vi "Set Rate (RPM).vi"(8 "error in (no error)":errorcluster, 10 "Rate (RPM)":dbl, 11 "Comp Motors with Encoders in":refnum<class "Comp Motors with Encoders.lvclass">) -> (0 "error out":errorcluster, 3 "Comp Motors with Encoders out":refnum<class "Comp Motors with Encoders.lvclass">)   [LabVIEW 2014, in "Comp Motors with Encoders.lvlib" / "Comp Motors with Encoders.lvclass"]
uses:
  Comp Motors with Encoders.lvclass
  Comp Motors with Encoders.lvclass/Comp Motors with Encoders.ctl
  Robot/Motor with Encoders/Motors with Encoders Class/Motors with Encoders.lvclass
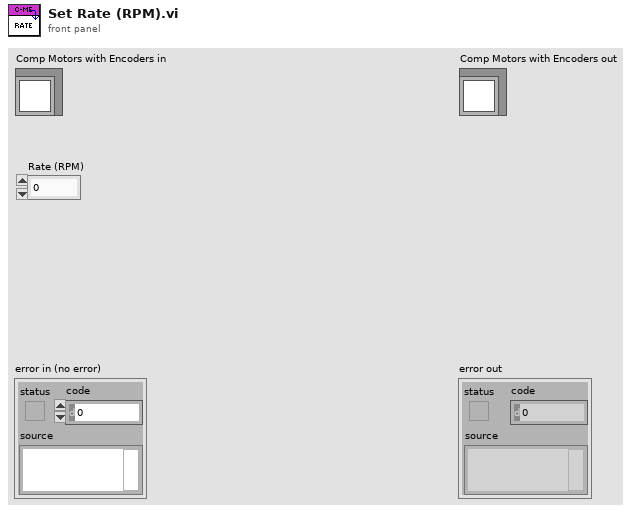
[diagram p1: front panel]
types:
  T1 = enum16{"Critical", "Error", "Warning", "Informational", "Debug"}
  T2 = typedef "WPI_MotorControlDeviceRef.ctl" = cluster{"DeviceStatus":errorcluster, "Type":T3, "PWM":cluster{"Controller":T4, "PWM Channel":T5, "DeadBand":T6}, "CAN":cluster{"Device Number":u8, "Control Mode":T7, "Semaphore":T8, "Max Vout":dbl, "TalonSRX Control Mode":T9}, "Invert":bool, "TransformRef":T10, "InvTransformRef":T10}
  T3 = typedef "WPI_MotorControlType.ctl" = enum16{"PWM", "CAN", "CANTalonSRX"}
  T4 = typedef "FPGA_TypedefDigitalModule.ctl" = enum16{"Controller 1"}
  T5 = typedef "FPGA_DIOPWMChannel.ctl" = enum8{"PWM 0", "PWM 1", "PWM 2", "PWM 3", "PWM 4", "PWM 5", "PWM 6", "PWM 7", "PWM 8", "PWM 9", "PWM MXP 0", "PWM MXP 1", "PWM MXP 2", "PWM MXP 3", "PWM MXP 4", "PWM MXP 5", "PWM MXP 6", "PWM MXP 7", "PWM MXP 8", "PWM MXP 9", "Invalid"}
  T6 = typedef "WPI_PWMDeadband.ctl" = cluster{"Name":string, "maxPositivePwm":i32, "minPositivePwm":i32, "centerPwm":i32, "maxNegativePwm":i32, "minNegativePwm":i32, "angularRange":u16}
  T7 = typedef "WPI_CANJaguar_ControlMode.ctl" = enum8{"Percent VBus", "Current", "Speed", "Position", "Voltage"}
  T8 = typedef "Semaphore RefNum" = refnum<k1>
  T9 = typedef "WPI_CANTalonSRX_APIControlMode.ctl" = enum8{"Percent VBus", "Speed", "Position", "Slave", "Unchanged / Invalid"}
  T10 = typedef "WPI_PWMTransform_ConPane.ctl" = refnum<vi>
  T11 = typedef "Motors with Encoders.lvlib/Motors with Encoders.lvclass/Motors with Encoders State.ctl" = cluster{"Forward Switch":bool, "Reverse Switch":bool, "Measured RPM":dbl, "Distance (in)":dbl, "Setpoint RPM":dbl, "Encoder Count":i64, "Home Count":i64, "Config":T12}
  T12 = typedef "Motors with Encoders.lvlib/Motors with Encoders.lvclass/Motors with Encoders Config.ctl" = cluster{"Counts  Per Revolution":u32, "Invert Encoder Direction":bool, "Diameter of Revolution":dbl, "Max RPM":dbl, "Encoder Control":bool}
  T13 = typedef "WPI_CANTalonSRX_GlobalStatus.ctl" = cluster{"Applied Throttle":dbl, "Module Enabled":bool, "CAN Error":errorcluster, "Closed Loop Error":dbl, "Forward Limit Switch Closed":bool, "Reverse Limit Switch Closed":bool, "Sensor Position":dbl, "Sensor Velocity":dbl, "Current":dbl, "Sticky Fault - Over Temp":bool, "Sticky Fault - Under Voltage":bool, "Sticky Fault - Forward Limit":bool, "Sticky Fault - Reverse Limit":bool, "Sticky Fault - Forward Soft Limit":bool, "Sticky Fault - Reverse Soft Limit":bool, "Brake is Enabled":bool, "Encoder Position":dbl, "Encoder Velocity":dbl, "Encoder Index Count":dbl, "Encoder A Pin State":bool, "Encoder B Pin State":bool, "Encoder Index Pin State":bool, "Analog In":dbl, "Analog In Velocity":dbl, "Temperature (C)":dbl, "Battery Voltage":dbl}
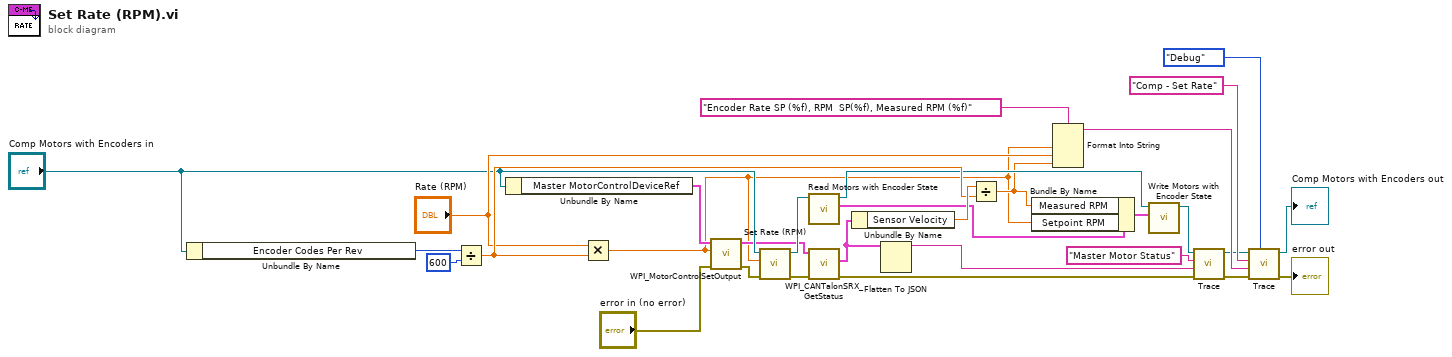
[diagram p0: block diagram]
diagram:
  n1 = Unbundle By Name("Comp Motors with Encoders in") -> ("Encoder Codes Per Rev"=w17:u16)
  n2 = Divide(x=w17, y=u16 600) -> (x/y=w13:dbl)
  n3 = Unbundle By Name("Comp Motors with Encoders in") -> ("Master MotorControlDeviceRef"=w30:T2)
  n4 = Multiply(x="Rate (RPM)", y=w13) -> (x*y=w1:dbl)
  n5 = call <vilib>:"WPI_MotorControlSetOutput.vi"("error in (no error)"="error in (no error)", "Output"=w1, "MotorControlDevRef"=w30) -> ("error out"=w2:errorcluster, "MotorControlDevRef"=w3:T2)  [unwired: 6 in, 1 out]
  n6 = call-parent "Set Rate (RPM).vi"("error in (no error)"=w2, "Rate (RPM)"=w1, "Motors with Encoders in"="Comp Motors with Encoders in") -> ("error out"=w23:errorcluster, "Motors with Encoders out"=w12:refnum<class "Comp Motors with Encoders.lvclass">)  [unwired: 7 in]
  n7 = call-dynamic "Read Motors with Encoder State.vi"("Motors with Encoders in"=w12) -> ("Motors with Encoder State"=w9:T11, "Motors with Encoders out"=w11:refnum<class "Comp Motors with Encoders.lvclass">)  [unwired: 8 in, 1 out]
  n8 = call <vilib>:"WPI_CANTalonSRX_GetStatus.vi"("error in (no error)"=w23, "CAN Talon SRX Ref"=w3) -> ("error out"=w22:errorcluster, "Talon SRX Status"=w15:T13)  [unwired: 7 in, 1 out]
  n9 = Unbundle By Name(w15) -> ("Sensor Velocity"=w14:dbl)
  n10 = Flatten To JSON(anything=w15) -> (JSON string=w19:string)  [unwired: 2 in, 1 out]
  n11 = Divide(x=w14, y=w13) -> (x/y=w7:dbl)
  n12 = Bundle By Name(cluster=w9, "Measured RPM"=w7, "Setpoint RPM"=w1) -> (w8:T11)
  n13 = Format Into String(format string="Encoder Rate SP (%f), RPM  SP(%f), Measured RPM (%f)", w1, "Rate (RPM)", w7) -> (resulting string=w24:string)  [unwired: 2 in, 1 out]
  n14 = call-dynamic "Write Motors with Encoder State.vi"("Motors with Encoder State"=w8, "Motors with Encoders in"=w11) -> ("Motors with Encoders out"=w10:refnum<class "Comp Motors with Encoders.lvclass">)  [unwired: 8 in, 1 out]
  n15 = call-dynamic "Trace.vi"("error in (no error)"=w22, "System Message"=w19, "System Action"="Master Motor Status", "System Actor in"=w10) -> ("error out"=w21:errorcluster, "System Actor out"=w20:refnum<class "Comp Motors with Encoders.lvclass">)  [unwired: 6 in]
  n16 = call-dynamic "Trace.vi"("Trace Level"=T1."Debug", "error in (no error)"=w21, "System Message"=w24, "System Action"="Comp - Set Rate", "System Actor in"=w20) -> ("error out"=→"error out":errorcluster, "System Actor out"=→"Comp Motors with Encoders out":refnum<class "Comp Motors with Encoders.lvclass">)  [unwired: 5 in]
